vi "水样测试.vi"(10 "数据标记表":string(combo)="N", 11 "水样测试时间":dbl=1.0) -> ()   [LabVIEW 2016, in "斯坦道多参数.lvlib"]
panel:
  out "运行状态":u16(ring) items=["空闲", "水样测试", "标样核查"]
  out "多参数运行日志":string
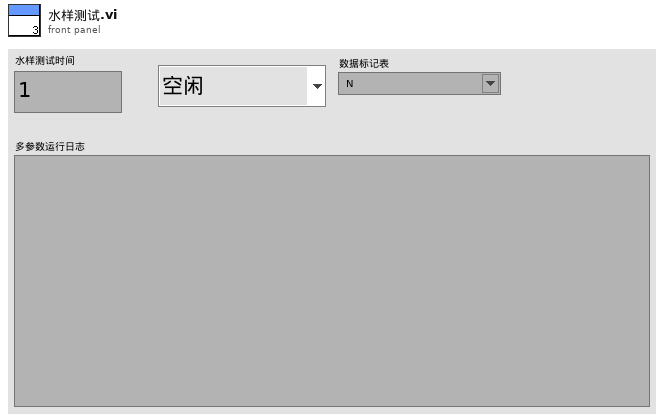
[diagram p1: front panel]
types:
  T1 = cluster{"因子编码":string, "单位":string, "标样参考值":sgl, "水样数据时间":timestamp, "水样实测值":sgl, "水样数据标识":string, "探头温度":sgl}
  T2 = cluster{"温度测量值":sgl, "DO%":sgl, "DOmg/L":sgl, "温度偏移修正值":sgl}
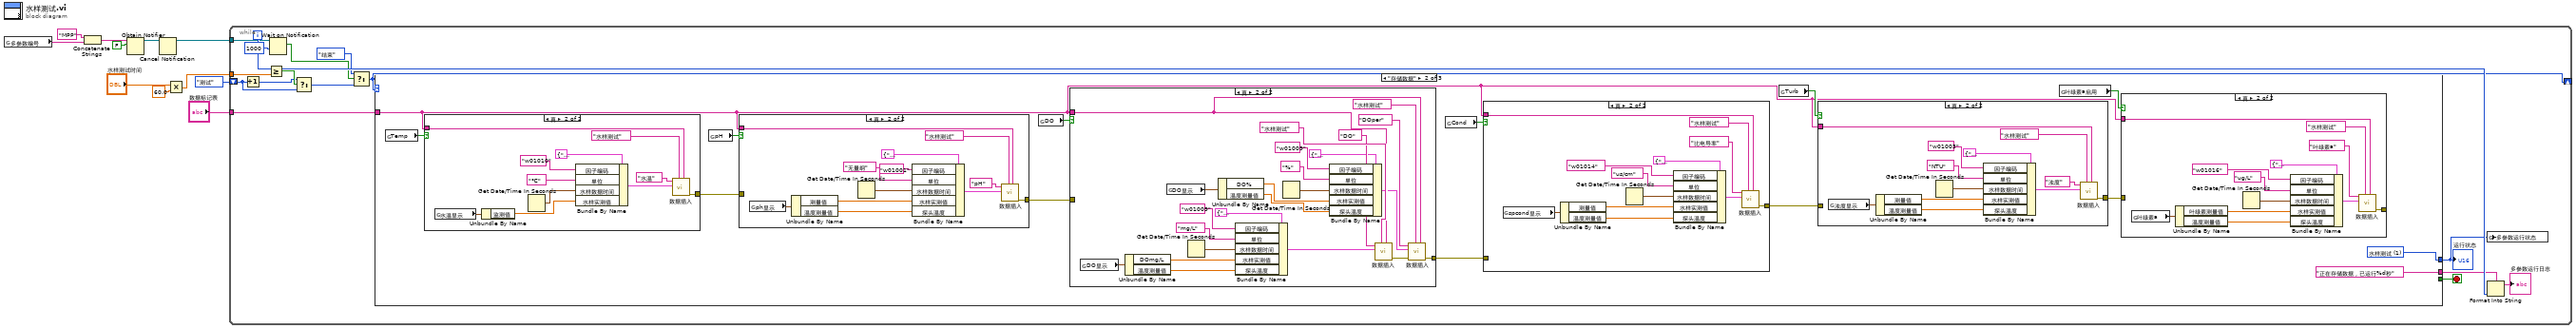
[diagram p0: block diagram]
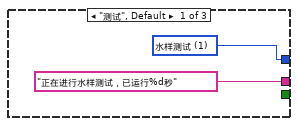
[diagram p2: hidden frame]
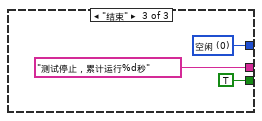
[diagram p9: hidden frame]
diagram:
  n1 = global read "多参数全局变量.vi" "多参数编号"() -> (w1:string)
  n2 = Concatenate Strings("MPP" ("名称（未命名）"), w1) -> (w2:string)
  n3 = Obtain Notifier(name (unnamed)=w2, notification data type=FALSE) -> (notifier out=w5:refnum<notifier>)  [unwired: 2 in, 2 out]
  n4 = Cancel Notification(0:w5) -> (8:w4:refnum<notifier>)  [unwired: 1 in, 2 out]
  n5 = Multiply(x="水样测试时间", y=60.0) -> (x*y=w9:dbl)
  n6 = while {
    tunnel: w9 -> [w27]
    shift-right: [w14] -> _
    shift-left: enum16{"测试", "存储数据", "结束"}."测试" ("枚举") -> [w21]
    tunnel: w4 -> [w19]
    tunnel: "数据标记表" -> [w13]
    i -> [w25]
    stop <- w26 stop-if-true
    n7 = Increment(x=w21) -> (x+1=w20:enum16{"测试", "存储数据", "结束"})
    n8 = Greater Or Equal?(x=w25, y=w27) -> (x >= y?=w22:bool)
    n9 = Wait on Notification(notifier=w19, timeout in ms (-1)=1000 ("超时毫秒(-1)")) -> (notification=w17:bool)  [unwired: 2 in, 3 out]
    n10 = Select(t=w20, s=w22, f=w21) -> (s? t:f=w15:enum16{"测试", "存储数据", "结束"})
    n11 = Select(t=enum16{"测试", "存储数据", "结束"}."结束" ("枚举"), s=w17, f=w15) -> (s? t:f=w14:enum16{"测试", "存储数据", "结束"})
    n12 = case shown="\"存储数据\"" w14 {
      tunnel: [_ _ TRUE] -> w26
      tunnel: ["正在进行水样测试，已运行%d秒" ("格式字符串") "正在存储数据，已运行%d秒" ("格式字符串") "测试停止，累计运行%d秒" ("格式字符串")] -> w24
      tunnel: [w28 w31 w126] -> w12
      tunnel: w13 -> [_ w30 _]
      frame "测试", Default {
        w28 = u16 1 items=["空闲", "水样测试", "标样核查"] ("多参数运行状态")
      }
      frame "存储数据" {
        w31 = u16 1 items=["空闲", "水样测试", "标样核查"] ("多参数运行状态")
        n13 = global read "断电保存变量.vi" "Temp"() -> (w38:bool)
        n14 = case shown="真" w38 {
          tunnel: [_ w118] -> w33
          tunnel: w30 -> [_ w117]
          frame False {
          }
          frame True {
            n15 = global read "多参数全局变量.vi" "水温显示"() -> (w116:cluster{"CH":u16, "监测值":dbl, "温度偏移修正值":sgl})
            n16 = Unbundle By Name(w116) -> ("监测值"=w115:dbl)
            n17 = Get Date/Time In Seconds() -> (seconds since 1Jan1904=w124:timestamp)
            n18 = Bundle By Name(cluster=T1 {"因子编码"="w01003", "单位"="无量纲", "标样参考值"=0.0, "水样数据时间"=timestamp(0 s since 1904-01-01), "水样实测值"=0.0, "水样数据标识"="N", "探头温度"=0.0} ("data in"), "因子编码"="w01010", "单位"="℃", "水样数据时间"=w124, "水样实测值"=w115) -> (w123:T1)
            n19 = call "数据插入.vi"("数据标记表"=w117, "测量模式"="水样测试", "data in"=w123, "table输入"="水温") -> ("error out"=w118:errorcluster)  [unwired: 7 in]
          }
        }
        n20 = global read "断电保存变量.vi" "pH"() -> (w39:bool)
        n21 = case shown="真" w39 {
          tunnel: w33 -> [_ _]
          tunnel: [_ w107] -> w34
          tunnel: w30 -> [_ w106]
          frame False {
          }
          frame True {
            n22 = global read "多参数全局变量.vi" "ph显示"() -> (w105:cluster{"温度测量值":sgl, "测量值":sgl, "温度偏移修正值":sgl})
            n23 = Unbundle By Name(w105) -> ("测量值"=w104:sgl, "温度测量值"=w103:sgl)
            n24 = Get Date/Time In Seconds() -> (seconds since 1Jan1904=w112:timestamp)
            n25 = Bundle By Name(cluster=T1 {"因子编码"="w01003", "单位"="无量纲", "标样参考值"=0.0, "水样数据时间"=timestamp(0 s since 1904-01-01), "水样实测值"=0.0, "水样数据标识"="N", "探头温度"=0.0} ("data in"), "因子编码"="w01001", "单位"="无量纲", "水样数据时间"=w112, "水样实测值"=w104, "探头温度"=w103) -> (w113:T1)
            n26 = call "数据插入.vi"("数据标记表"=w106, "测量模式"="水样测试", "data in"=w113, "table输入"="pH") -> ("error out"=w107:errorcluster)  [unwired: 7 in]
          }
        }
        n27 = global read "断电保存变量.vi" "DO"() -> (w40:bool)
        n28 = case shown="真" w40 {
          tunnel: w34 -> [_ _]
          tunnel: [_ w95] -> w35
          tunnel: w30 -> [_ w93]
          frame False {
          }
          frame True {
            n29 = global read "多参数全局变量.vi" "DO显示"() -> (w84:T2)
            n30 = Unbundle By Name(w84) -> ("DOmg/L"=w83:sgl, "温度测量值"=w82:sgl)
            n31 = global read "多参数全局变量.vi" "DO显示"() -> (w81:T2)
            n32 = Get Date/Time In Seconds() -> (seconds since 1Jan1904=w101:timestamp)
            n33 = Unbundle By Name(w81) -> ("DO%"=w88:sgl, "温度测量值"=w86:sgl)
            n34 = Bundle By Name(cluster=T1 {"因子编码"="w01003", "单位"="无量纲", "标样参考值"=0.0, "水样数据时间"=timestamp(0 s since 1904-01-01), "水样实测值"=0.0, "水样数据标识"="N", "探头温度"=0.0} ("data in"), "因子编码"="w01009", "单位"="mg/L", "水样数据时间"=w101, "水样实测值"=w83, "探头温度"=w82) -> (w100:T1)
            n35 = Get Date/Time In Seconds() -> (seconds since 1Jan1904=w89:timestamp)
            n36 = Bundle By Name(cluster=T1 {"因子编码"="w01003", "单位"="无量纲", "标样参考值"=0.0, "水样数据时间"=timestamp(0 s since 1904-01-01), "水样实测值"=0.0, "水样数据标识"="N", "探头温度"=0.0} ("data in"), "因子编码"="w01009", "单位"="%", "水样数据时间"=w89, "水样实测值"=w88, "探头温度"=w86) -> (w85:T1)
            n37 = call "数据插入.vi"("数据标记表"=w93, "测量模式"="水样测试", "data in"=w100, "table输入"="DO") -> ("error out"=w80:errorcluster)  [unwired: 7 in]
            n38 = call "数据插入.vi"("数据标记表"=w93, "测量模式"="水样测试", "error in (no error)"=w80, "data in"=w85, "table输入"="DOper") -> ("error out"=w95:errorcluster)  [unwired: 6 in]
          }
        }
        n39 = global read "断电保存变量.vi" "Cond"() -> (w41:bool)
        n40 = case shown="真" w41 {
          tunnel: w35 -> [_ _]
          tunnel: [_ w72] -> w36
          tunnel: w30 -> [_ w71]
          frame False {
          }
          frame True {
            n41 = global read "多参数全局变量.vi" "spcond显示"() -> (w70:cluster{"温度测量值":sgl, "测量值":sgl, "温度偏移修正值":sgl})
            n42 = Unbundle By Name(w70) -> ("测量值"=w69:sgl, "温度测量值"=w68:sgl)
            n43 = Get Date/Time In Seconds() -> (seconds since 1Jan1904=w77:timestamp)
            n44 = Bundle By Name(cluster=T1 {"因子编码"="w01003", "单位"="无量纲", "标样参考值"=0.0, "水样数据时间"=timestamp(0 s since 1904-01-01), "水样实测值"=0.0, "水样数据标识"="N", "探头温度"=0.0} ("data in"), "因子编码"="w01014", "单位"="us/cm", "水样数据时间"=w77, "水样实测值"=w69, "探头温度"=w68) -> (w78:T1)
            n45 = call "数据插入.vi"("数据标记表"=w71, "测量模式"="水样测试", "data in"=w78, "table输入"="比电导率") -> ("error out"=w72:errorcluster)  [unwired: 7 in]
          }
        }
        n46 = global read "断电保存变量.vi" "Turb"() -> (w42:bool)
        n47 = case shown="真" w42 {
          tunnel: w36 -> [_ _]
          tunnel: [_ w60] -> w37
          tunnel: w30 -> [_ w59]
          frame False {
          }
          frame True {
            n48 = global read "多参数全局变量.vi" "浊度显示"() -> (w58:cluster{"温度测量值":sgl, "测量值":sgl, "温度偏移修正值":sgl})
            n49 = Unbundle By Name(w58) -> ("测量值"=w57:sgl, "温度测量值"=w56:sgl)
            n50 = Get Date/Time In Seconds() -> (seconds since 1Jan1904=w66:timestamp)
            n51 = Bundle By Name(cluster=T1 {"因子编码"="w01003", "单位"="无量纲", "标样参考值"=0.0, "水样数据时间"=timestamp(0 s since 1904-01-01), "水样实测值"=0.0, "水样数据标识"="N", "探头温度"=0.0} ("data in"), "因子编码"="w01003", "单位"="NTU", "水样数据时间"=w66, "水样实测值"=w57, "探头温度"=w56) -> (w65:T1)
            n52 = call "数据插入.vi"("数据标记表"=w59, "测量模式"="水样测试", "data in"=w65, "table输入"="浊度") -> ("error out"=w60:errorcluster)  [unwired: 7 in]
          }
        }
        n53 = global read "断电保存变量.vi" "叶绿素a启用"() -> (w43:bool)
        n54 = case shown="真" w43 {
          tunnel: w37 -> [_ _]
          tunnel: [_ w46] -> _
          tunnel: w30 -> [_ w45]
          frame False {
          }
          frame True {
            n55 = global read "禹山过程全局变量.vi" "叶绿素a"() -> (w44:cluster{"温度测量值":sgl, "叶绿素测量值":sgl, "错误标志":u16})
            n56 = Unbundle By Name(w44) -> ("叶绿素测量值"=w53:sgl, "温度测量值"=w51:sgl)
            n57 = Get Date/Time In Seconds() -> (seconds since 1Jan1904=w54:timestamp)
            n58 = Bundle By Name(cluster=T1 {"因子编码"="w01003", "单位"="无量纲", "标样参考值"=0.0, "水样数据时间"=timestamp(0 s since 1904-01-01), "水样实测值"=0.0, "水样数据标识"="N", "探头温度"=0.0} ("data in"), "因子编码"="w01016", "单位"="ug/L", "水样数据时间"=w54, "水样实测值"=w53, "探头温度"=w51) -> (w49:T1)
            n59 = call "数据插入.vi"("数据标记表"=w45, "测量模式"="水样测试", "data in"=w49, "table输入"="叶绿素a") -> ("error out"=w46:errorcluster)  [unwired: 7 in]
          }
        }
      }
      frame "结束" {
        w126 = u16 0 items=["空闲", "水样测试", "标样核查"] ("多参数运行状态")
      }
    }
    "运行状态" <- w12
    n60 = global write "多参数全局变量.vi" "多参数运行状态"(w12) -> ()
    n61 = Format Into String(format string=w24, w25) -> (resulting string=→"多参数运行日志":string)  [unwired: 2 in, 1 out]
  }
